vi "gl_Funct imaging UI.vi"() -> ()   [LabVIEW 2020]
panel:
  in  "New Experiment folder path":path
  in  "\"Funct img\" bring to front":bool
  in  "\"Funct img\" window is open":bool
  in  "\"Funct img\" close window":bool
  # "<--- not used"
  # "Used by the viewer when it is already open, to receive the new path of the dataset generated by a consecutive functional acquisition."
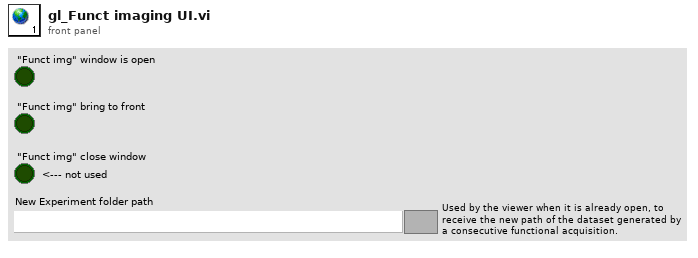
[diagram p1: front panel]
diagram:
